vi "SaveFile.vi"(9 "数据":string[][](array[string]), 10 "文件头":string[](array[string]), 11 "文件路径":path) -> (3 "Success":bool)   [LabVIEW 2011]
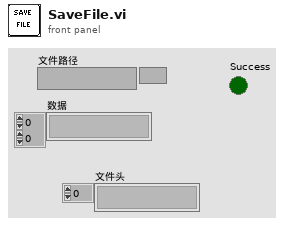
[diagram p1: front panel]
types:
  T1 = enum16{"open", "replace", "create", "open or create", "replace or create", "replace or create with confirmation"}
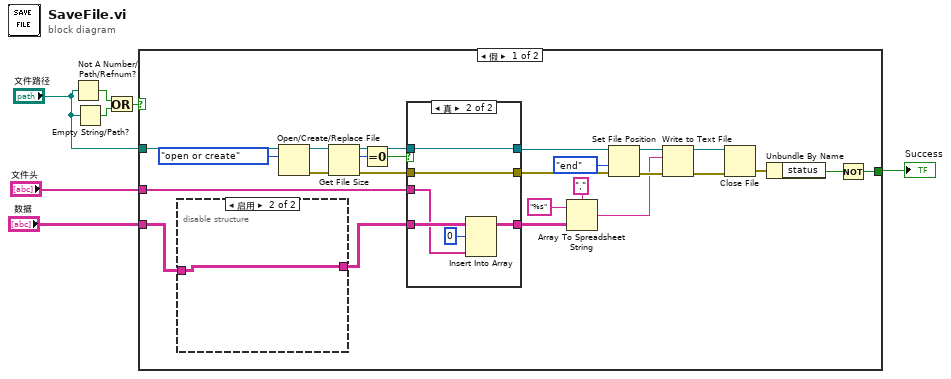
[diagram p0: block diagram]
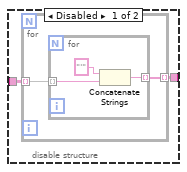
[diagram p2: hidden frame]
diagram:
  n1 = Not A Number/Path/Refnum?(number/path/refnum="文件路径") -> (NaN/Path/Refnum?=w7:bool)
  n2 = Empty String/Path?(string/path="文件路径") -> (empty?=w6:bool)
  n3 = Or(x=w7, y=w6) -> (x .or. y?=w5:bool)
  n4 = case shown="假" w5 {
    tunnel: "文件路径" -> [w32 _]
    tunnel: "文件头" -> [w24 _]
    tunnel: "数据" -> [w23 _]
    tunnel: [w9 _] -> w1
    frame False {
      n5 = disable-structure shown="启用" {
        disable-tunnel: w23 -> [w34 w40]
        disable-tunnel: [w33 w40] -> w22
        frame Disabled {
          n6 = for {
            tunnel: w34 -> [w36] mode=indexing
            tunnel: [w35] -> w33 mode=indexing
            n7 = for {
              tunnel: w36 -> [w39] mode=indexing
              tunnel: [w37] -> w35 mode=indexing
              n8 = Concatenate Strings("'" ("字符串"), w39) -> (w37:string)
            }
          }
        }
        frame Enabled {
        }
      }
      n9 = Open/Create/Replace File(file path (use dialog)=w32, operation (0:open)=T1."open or create" ("操作(0:open)")) -> (refnum out=w30:refnum<file>, error out=w29:errorcluster)  [unwired: 4 in, 1 out]
      n10 = Get File Size(file=w30, error in=w29) -> (refnum out=w26:refnum<file>, size (in bytes)=w28:i64, 0:w25:errorcluster)
      n11 = Equal To 0?(x=w28) -> (x = 0?=w27:bool)
      n12 = case shown="真" w27 {
        tunnel: w26 -> [w42 w45]
        tunnel: w25 -> [w41 w44]
        tunnel: w24 -> [_ w48]
        tunnel: w22 -> [w43 w49]
        tunnel: [w43 w46] -> w20
        tunnel: [w42 w45] -> w19
        tunnel: [w41 w44] -> w18
        frame False {
        }
        frame True {
          n13 = Insert Into Array(array=w49, index (row)=0 ("索引 (行)"), new element=w48) -> (w46:string[][])  [unwired: 1 in]
        }
      }
      n14 = Array To Spreadsheet String(delimiter (Tab)="," ("分隔符(Tab)"), array=w20, 3:"%s" ("格式字符串")) -> (spreadsheet string=w14:string)
      n15 = Set File Position(refnum=w19, from (0:start)=enum16{"start", "end", "current"}."end" ("自（0:起始）"), error in=w18) -> (refnum out=w16:refnum<file>, error out=w15:errorcluster)  [unwired: 1 in]
      n16 = Write to Text File(file (use dialog)=w16, text=w14, error in=w15) -> (refnum out=w12:refnum<file>, error out=w13:errorcluster)  [unwired: 1 in, 1 out]
      n17 = Close File(refnum=w12, error in=w13) -> (error out=w11:errorcluster)  [unwired: 1 out]
      n18 = Unbundle By Name(w11) -> ("status"=w10:bool)
      n19 = Not(x=w10) -> (.not. x?=w9:bool)
    }
    frame True {
    }
  }
  "Success" <- w1
